vi "Read Column.vi"(8 "error in (no error)":errorcluster, 11 "2D Array in":refnum<class "2D Array.lvclass">) -> (0 "error out":errorcluster, 2 "Column":i32, 3 "2D Array out":refnum<class "2D Array.lvclass">)   [LabVIEW 2019, in "2D Array.lvclass"]
uses:
  2D Array.lvclass
  2D Array.lvclass/2D Array.ctl
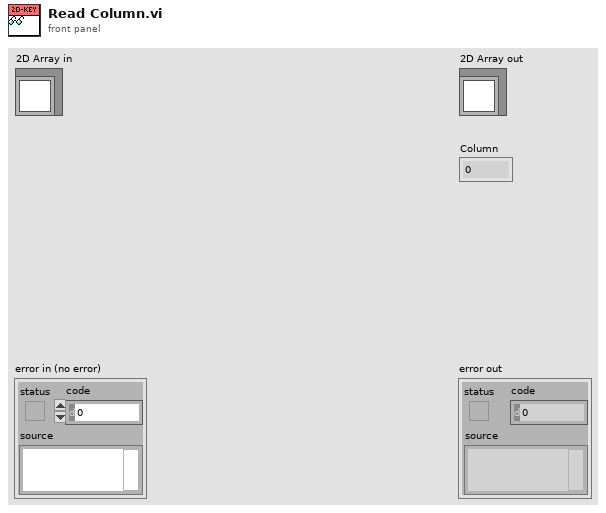
[diagram p1: front panel]
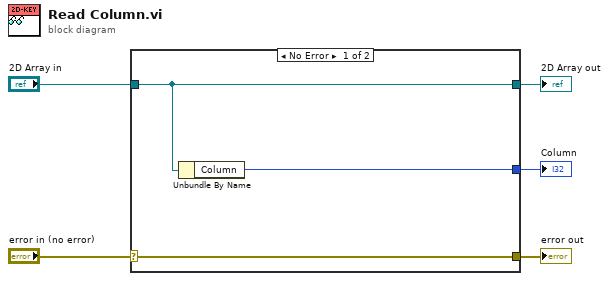
[diagram p0: block diagram]
diagram:
  n1 = case shown="No Error" "error in (no error)" {
    selector: "error in (no error)" -> [w8 w9]
    tunnel: [w8 w9] -> w4
    tunnel: [w7 w10] -> w2
    tunnel: "2D Array in" -> [w7 w10]
    tunnel: [w6 _] -> w1
    frame No Error {
      n2 = Unbundle By Name(w7) -> ("Column"=w6:i32)
    }
    frame Error {
    }
  }
  "error out" <- w4
  "2D Array out" <- w2
  "Column" <- w1
